vi "gesture recognition.vi"() -> ()   [LabVIEW 2020]
uses:
  <vilib>/Instr/_visa.llb/VISA Configure Serial Port (Instr).vi
panel:
  out "String":string
  in  "STOP":bool
  out "error out":errorcluster
  # "Move Your Hand To Express"
  # "Move Your Hand To Express"
  # "COMMAND READING...."
  # "STOP"
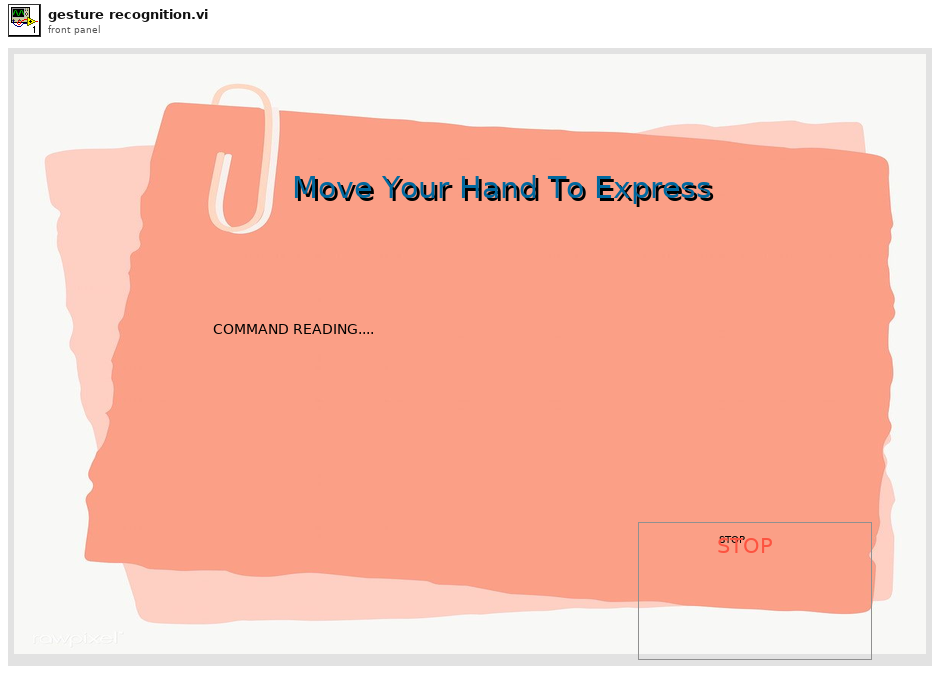
[diagram p1: front panel]
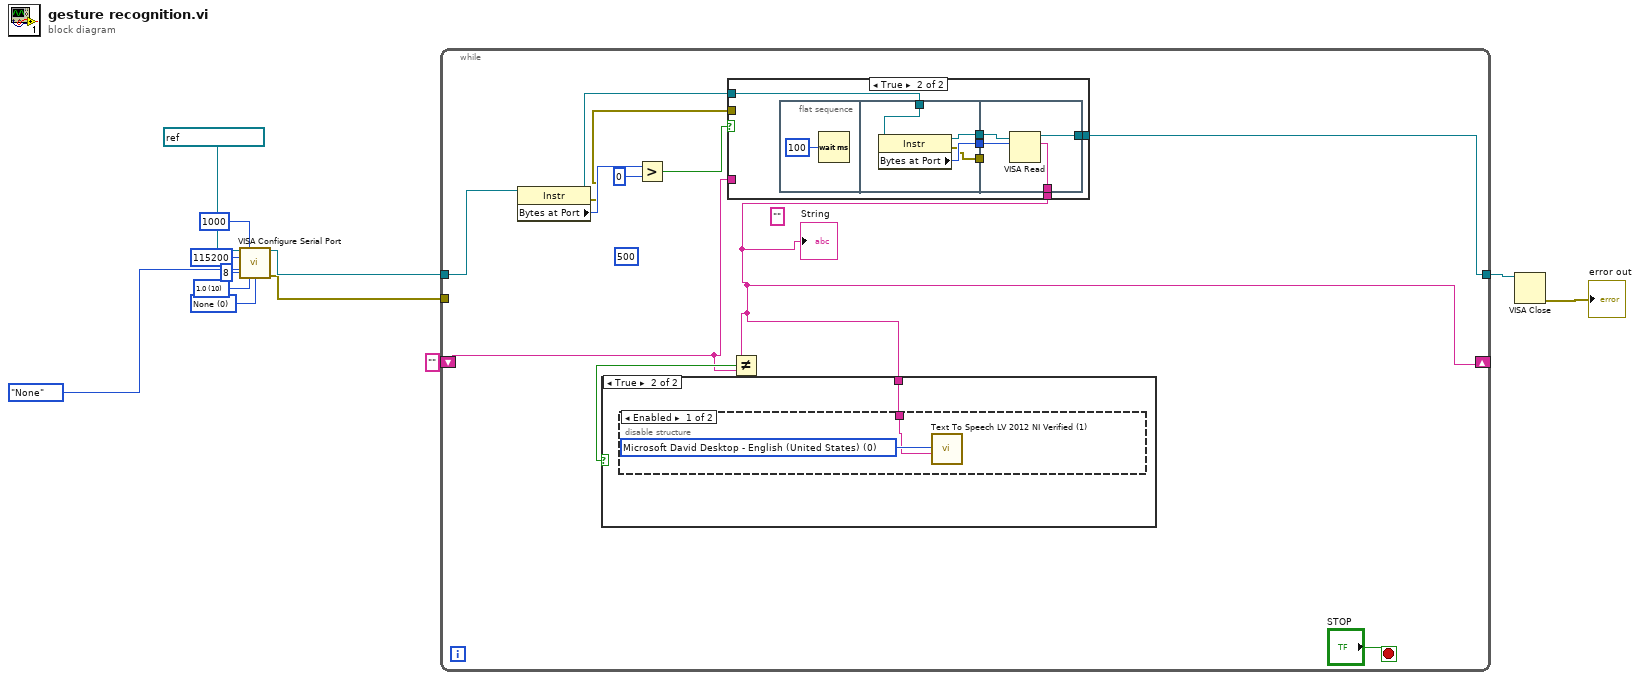
[diagram p0: block diagram]
diagram:
  w7 = u16 0 items=["None", "XON/XOFF", "RTS/CTS", "XON/XOFF & RTS/CTS", "DTR/DSR", "XON/XOFF & DTR/DSR"] ("flow control (0:none)")
  w8 = u16 10 items=["1.0"=10, "1.5"=15, "2.0"=20] ("stop bits (10: 1 bit)")
  n1 = call-poly "VISA Configure Serial Port"("VISA resource name"=refnum<visa-resource-name> "COM3", "timeout (10sec)"=u32 1000, "baud rate (9600)"=u32 115200, "data bits (8)"=u16 8, "parity (0:none)"=enum16{"None", "Odd", "Even", "Mark", "Space"}."None", "stop bits (10: 1 bit)"=w8, "flow control (0:none)"=w7) -> ("VISA resource name out"=w5:refnum<visa-resource-name>, "error out"=w4:errorcluster)  [unwired: 7 in]
  n2 = while {
    tunnel: [w14] -> w3
    tunnel: w5 -> [w21]
    tunnel: w4 -> [_]
    shift-right: [w15] -> _
    shift-left: "" ("read buffer") -> [w13]
    stop <- "STOP" stop-if-true
    (unwired) "" ("read buffer")
    (unwired) u32 500 ("byte count")
    n3 = property class="Instr"(reference=w21) -> (reference out=w16:refnum<visa-resource-name>, error out=w17:errorcluster, "Bytes at Port"=w20:u32)  [unwired: 1 in]
    n4 = Greater?(x=w20, y=u32 0) -> (0:w18:bool)
    n5 = case shown="True" w18 {
      tunnel: w17 -> [_ _]
      tunnel: w16 -> [w25 w31]
      tunnel: [w24 w28] -> w15
      tunnel: [w25 w27] -> w14
      tunnel: w13 -> [w24 _]
      frame False {
      }
      frame True {
        n6 = flat-sequence {
          tunnel: w31 -> [w36]
          tunnel: [w35] -> w30
          tunnel: [w34] -> w29
          tunnel: [w33] -> w26
          tunnel: w30 -> [w40]
          tunnel: w29 -> [w39]
          tunnel: [w38] -> w28
          tunnel: [w37] -> w27
          tunnel: w26 -> [_]
          frame #0 {
            n7 = Wait (ms)(milliseconds to wait=u32 100) -> ()  [unwired: 1 out]
          }
          frame #1 {
            n8 = property class="Instr"(reference=w36) -> (reference out=w34:refnum<visa-resource-name>, error out=w33:errorcluster, "Bytes at Port"=w35:u32)  [unwired: 1 in]
          }
          frame #2 {
            n9 = VISA Read(VISA resource name=w39, byte count=w40) -> (VISA resource name out=w37:refnum<visa-resource-name>, read buffer=w38:string)  [unwired: 1 in, 2 out]
          }
        }
      }
    }
    "String" <- w15
    n10 = Not Equal?(x=w15, y=w13) -> (x != y?=w23:bool)
    n11 = case shown="True" w23 {
      tunnel: w15 -> [_ w41]
      frame False {
      }
      frame True {
        n12 = disable-structure shown="Enabled" {
          disable-tunnel: w41 -> [w42 _]
          frame Enabled {
            w43 = 0 items=["Microsoft David Desktop - English (United States)", "Microsoft Zira Desktop - English (United States)", ""] ("Choose a Voice")
            n13 = call "Text To Speech LV 2012 NI Verified (1).vi"("Text To Be Spoken"=w42, "Choose a Voice"=w43) -> ()  [unwired: 8 in, 2 out]
          }
          frame Disabled {
          }
        }
      }
    }
  }
  n14 = VISA Close(VISA resource name=w3) -> (error out=→"error out":errorcluster)  [unwired: 1 in]
